vi "Unconfigure.vi"(3 "entrée d'erreur (pas d'erreur)":errorcluster caption="error in", 5 "ref in":refnum<k7>) -> (0 "sortie d'erreur":errorcluster caption="error out", 2 "ref out":refnum<k7>)   [LabVIEW 2010]
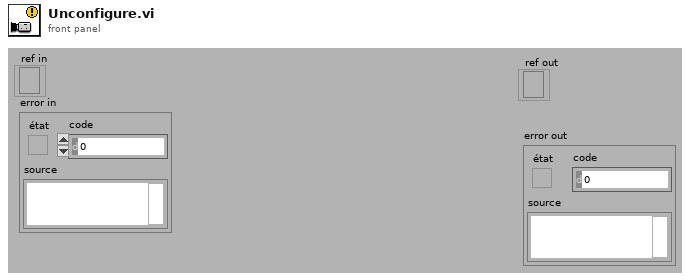
[diagram p1: front panel]
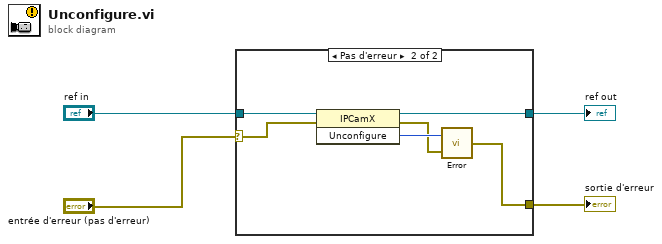
[diagram p0: block diagram]
diagram:
  n1 = case shown="Pas d'erreur" "entrée d'erreur (pas d'erreur)" {
    selector: "entrée d'erreur (pas d'erreur)" -> [w5 w11]
    tunnel: [w6 w10] -> w4
    tunnel: "ref in" -> [w6 w12]
    tunnel: [w5 w7] -> w2
    frame Error {
    }
    frame No Error {
      n2 = invoke class="IPCamX" method="Unconfigure"(reference=w12, error in=w11) -> (reference out=w10:refnum<k7>, error out=w8:errorcluster, "Unconfigure"=w9:i32)  [unwired: 1 in]
      n3 = call "Error.vi"("error in"=w8, "code"=w9) -> ("error out"=w7:errorcluster)
    }
  }
  "sortie d'erreur" <- w2
  "ref out" <- w4
